vi "Preview Action Queue.vi"(0 "action queue in":refnum<queue>, 11 "error in":errorcluster) -> (4 "action queue out":refnum<queue>, 8 "action elements":T1[](array[typedef]), 15 "error out":errorcluster)   [LabVIEW 2018, in "Springboard TLB`.lvlib" / "Actions.lvlib"]
doc: "Returns the element at the front of the queue without removing the element from the queue.\n\n<B>Input Parameters</B>\n\n<B>action queue in</B> is a reference to a queue. Use the Create Action Queue function to obtain a queue reference. \n\n<B>error in</B> describes error conditions that occur before this node runs. This input provides standard error in functionality.\n\n<B>Output Parameters</B>\n\n<B>action queue out</B> returns the reference to the queue unchanged. \n\n<B>action elements</B> returns actions enqueued into the system. \n\n<B>error out</B> contains error information. This output provides standard error out functionality."
uses:
  Actions.lvlib
  System Action Element.ctl
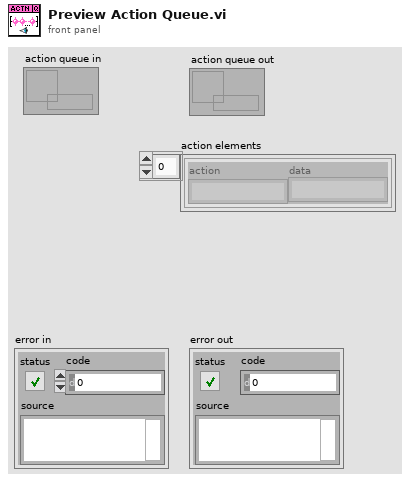
[diagram p1: front panel]
types:
  T1 = typedef "Springboard TLB`.lvlib/Actions.lvlib/System Action Element.ctl" = cluster{"action":string, "data":string}
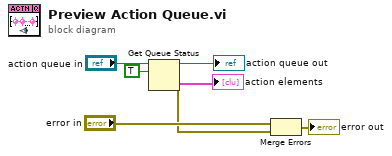
[diagram p0: block diagram]
diagram:
  n1 = Get Queue Status(queue="action queue in", return elements? (F)=TRUE) -> (queue out=→"action queue out":refnum<queue>, error out=w6:errorcluster, elements=→"action elements":T1[])  [unwired: 1 in, 5 out]
  n2 = Merge Errors("error in", w6) -> (→"error out":errorcluster)
